vi "Generate Maze.vi"(8 "error in (no error)":errorcluster, 9 "Height":i32, 10 "Width":i32, 11 "Intermediate Maze in":refnum<class "Intermediate MazeGen.lvclass">) -> (0 "error out":errorcluster, 2 "Maze":refnum<class "Maze.lvclass">, 3 "Intermediate Maze out":refnum<class "Intermediate MazeGen.lvclass">)   [LabVIEW 2020, in "Maze.lvlib" / "Intermediate MazeGen.lvclass"]
uses:
  Intermediate MazeGen.lvclass
  Maze/Maze.lvclass
  Position.ctl
  Direction.ctl
  MazeGen/MazeGen.lvclass
  Maze.lvlib
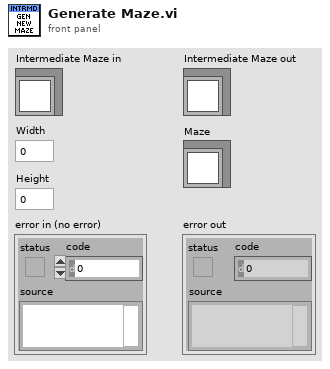
[diagram p1: front panel]
types:
  T1 = typedef "Maze.lvlib/Direction.ctl" = enum8{"East", "North", "West", "South"}
  T2 = typedef "Maze.lvlib/Position.ctl" = cluster{"S":i32, "E":i32}
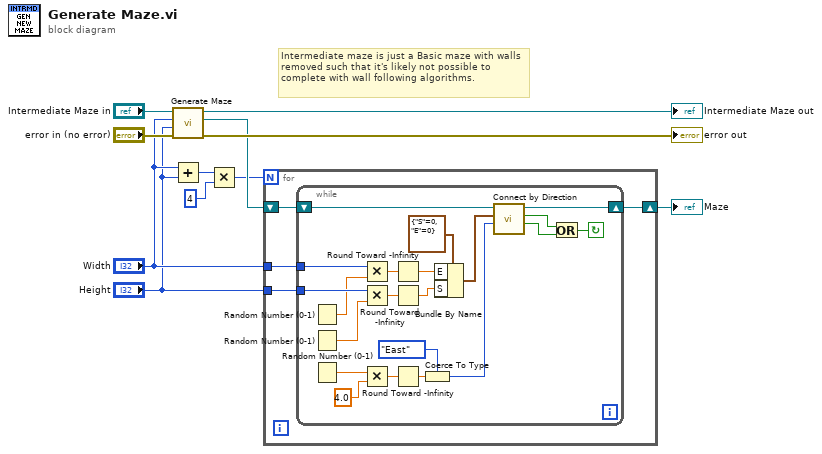
[diagram p0: block diagram]
diagram:
  # "Intermediate maze is just a Basic maze with walls removed such that it's likely not possible to complete with wall following algorithms."
  n1 = call-parent "Generate Maze.vi"("error in (no error)"="error in (no error)", "Height"="Height", "Width"="Width", "MazeGen in"="Intermediate Maze in") -> ("error out"=→"error out":errorcluster, "Maze"=w6:refnum<class "Maze.lvclass">, "MazeGen out"=→"Intermediate Maze out":refnum<class "Intermediate MazeGen.lvclass">)  [unwired: 5 in]
  n2 = Add(x="Width", y="Height") -> (x+y=w7:i32)
  n3 = Multiply(x=w7, y=4) -> (x*y=w2:i32)
  n4 = for {
    N: w2 -> [_]
    shift-right: [w14] -> w3
    shift-left: w6 -> [w15]
    tunnel: "Width" -> [w13]
    tunnel: "Height" -> [w12]
    n5 = while {
      shift-right: [w18] -> w14
      shift-left: w15 -> [w36]
      tunnel: w13 -> [w35]
      tunnel: w12 -> [w34]
      stop <- w17 continue-if-true
      n6 = Random Number (0-1)() -> (number: 0 to 1=w33:dbl)
      n7 = Random Number (0-1)() -> (number: 0 to 1=w32:dbl)
      n8 = Random Number (0-1)() -> (number: 0 to 1=w31:dbl)
      n9 = Multiply(x=w35, y=w33) -> (x*y=w29:dbl)
      n10 = Multiply(x=w34, y=w32) -> (x*y=w27:dbl)
      n11 = Multiply(x=w31, y=4.0) -> (x*y=w23:dbl)
      n12 = Round Toward -Infinity(1:w29) -> (0:w25:dbl)
      n13 = Round Toward -Infinity(1:w27) -> (0:w24:dbl)
      n14 = Round Toward -Infinity(1:w23) -> (0:w22:dbl)
      n15 = Coerce To Type(0:w22, 1:Direction."East" ("Direction")) -> (2:w20:T1)
      n16 = Bundle By Name(cluster=T2 {"S"=0, "E"=0} ("From"), "E"=w25, "S"=w24) -> (w26:T2)
      n17 = call "Connect by Direction.vi"("Direction"=w20, "From"=w26, "Maze in"=w36) -> ("Out of Bounds"=w16:bool, "Already Connected"=w19:bool, "Maze out"=w18:refnum<class "Maze.lvclass">)  [unwired: 5 in, 1 out]
      n18 = Or(x=w19, y=w16) -> (x .or. y?=w17:bool)
    }
  }
  "Maze" <- w3
